vi "Linear Fit PtByPt.vi"(0 "y":dbl format="%0.2f", 1 "initialize":bool, 7 "x":dbl format="%0.2f", 11 "sample length":i32=100) -> (4 "Best Linear Fit":dbl[](array[numeric]), 6 "slope":dbl format="%0.2f", 8 "intercept":dbl format="%0.2f", 10 "mse":dbl format="%0.2f", 15 "error":i32)   [LabVIEW 2020, in "NI_PtbyPt.lvlib"]
doc: "Finds the line values and the coefficients <B>slope</B> and <B>intercept</B>, using the least-squares solution, that describe the line that best represents the set of input data points specified by <B>sample length</B>."
uses:
  <vilib>/ptbypt/NI_PtbyPt.lvlib
  <vilib>/Analysis/NI_AALPro.lvlib
  <vilib>/Analysis/NI_AALBase.lvlib
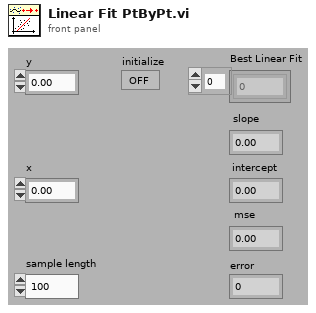
[diagram p1: front panel]
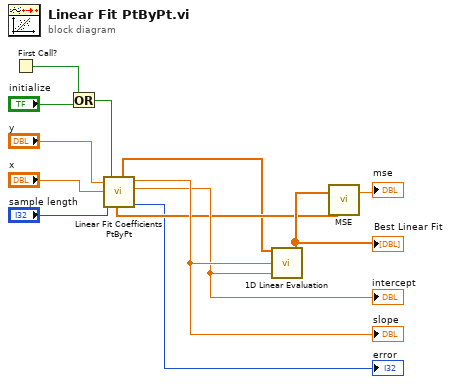
[diagram p0: block diagram]
diagram:
  n1 = First Call?() -> (First Call?: T/F=w1:bool)
  n2 = Or(x=w1, y="initialize") -> (x .or. y?=w2:bool)
  n3 = call <vilib>:"Linear Fit Coefficients PtByPt.vi"("y"="y", "x"="x", "sample length"="sample length", "initialize"=w2) -> ("History of x"=w6:dbl[], "History of y"=w8:dbl[], "slope"=w13:dbl, "intercept"=w12:dbl, "error"=→"error":i32)  [unwired: 2 in]
  "slope" <- w13
  "intercept" <- w12
  n4 = call <vilib>:"1D Linear Evaluation.vi"("offset"=w12, "scale"=w13, "X"=w6) -> ("Y[i]=X[i]*a+b"=w10:dbl[])  [unwired: 1 out]
  "Best Linear Fit" <- w10
  n5 = call <vilib>:"MSE.vi"("X Values"=w8, "Y Values"=w10) -> ("mse"=→"mse":dbl)  [unwired: 1 out]
